vi "Make Connections.vi"(8 "error in (no error)":errorcluster, 10 "relays to open":T1 {"position" items=["Open"=10, "Closed"=11]}, 11 "SLSC Switch in":refnum<class "SLSC Switch.lvclass">) -> (0 "error out":errorcluster, 3 "SLSC Switch out":refnum<class "SLSC Switch.lvclass">)   [LabVIEW 2015, in "SLSC Switch.lvclass"]
uses:
  SLSC Switch.lvclass
  slscsl/SwitchActionList.ctl
  slscsl/SwitchAction.ctl
  slscsl/RelayPosition.ctl
  SLSC Switch.lvclass/SLSC Switch.ctl
  Relay Interface/RelayInterface.lvclass
  slscsl/slscsl.lvclass
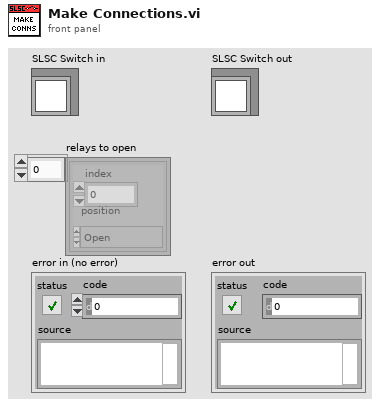
[diagram p1: front panel]
types:
  T1 = typedef "slscsl.lvclass/SwitchActionList.ctl" = T2[]
  T2 = typedef "slscsl.lvclass/SwitchAction.ctl" = cluster{"index":i32, "position":T3}
  T3 = typedef "slscsl.lvclass/RelayPosition.ctl" = i32
  T4 = typedef "slscsl.lvclass/RelayAction.ctl" = enum16{"Open Relay", "Close Relay"}
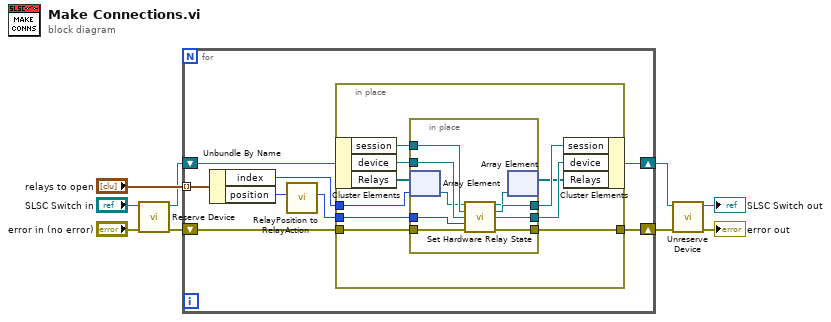
[diagram p0: block diagram]
diagram:
  n1 = call "Reserve Device.vi"("error in (no error)"="error in (no error)", "SLSC Switch in"="SLSC Switch in") -> ("error out"=w3:errorcluster, "SLSC Switch out"=w4:refnum<class "SLSC Switch.lvclass">)  [unwired: 8 in]
  n2 = for {
    tunnel: "relays to open" -> [w17] mode=indexing
    shift-right: [w10] -> w2
    shift-left: w4 -> [w12]
    shift-right: [w13] -> w1
    shift-left: w3 -> [w16]
    n3 = Unbundle By Name(w17) -> ("index"=w11:i32, "position"=w15:T3)
    n4 = call "RelayPosition to RelayAction.vi"("position"=w15) -> ("action"=w14:T4)  [unwired: 10 in]
    n5 = in-place {
      in-place-border: w16 -> [w27]
      in-place-border: w14 -> [w26]
      in-place-border: [w25] -> w13
      in-place-border: w11 -> [w19]
      n6 = in-place-cluster #1(w12) -> ("session"=w24:refnum<k21>, "device"=w23:refnum<k21>, "Relays"=w20:refnum<class "RelayInterface.lvclass">[])
      n7 = in-place {
        in-place-border: w27 -> [w36]
        in-place-border: w26 -> [w35]
        in-place-border: [w34] -> w25
        in-place-border: w24 -> [w33]
        in-place-border: w23 -> [w32]
        in-place-border: [w31] -> w22
        in-place-border: [w30] -> w21
        n8 = in-place-array #2(w20, w19) -> (w29:refnum<class "RelayInterface.lvclass">)
        n9 = call-dynamic "Set Hardware Relay State.vi"("RelayInterface in"=w29, "session in"=w33, "device in"=w32, "relay action (Close Relay)"=w35, "error in (no error)"=w36) -> ("RelayInterface out"=w28:refnum<class "RelayInterface.lvclass">, "session out"=w31:refnum<k21>, "device out"=w30:refnum<k21>, "error out"=w34:errorcluster)  [unwired: 7 in]
        n10 = in-place-array #2(w28) -> (w18:refnum<class "RelayInterface.lvclass">[])  [unwired: 1 out]
      }
      n11 = in-place-cluster #1("session"=w22, "device"=w21, "Relays"=w18) -> (w10:refnum<class "SLSC Switch.lvclass">)
    }
  }
  n12 = call "Unreserve Device.vi"("error in (no error)"=w1, "SLSC Switch in"=w2) -> ("error out"=→"error out":errorcluster, "SLSC Switch out"=→"SLSC Switch out":refnum<class "SLSC Switch.lvclass">)  [unwired: 8 in]
